vi "StatisticsFromArray.vi"(6 "Naverage":i32, 9 "input Ptot":dbl, 10 "input VAR":dbl[][](array[numeric]), 11 "Stat Vars":T1) -> (0 "STD":dbl[][](graph), 1 "MU":dbl[][](graph), 3 "VAR(n+1)":T1, 5 "std":dbl, 7 "mu":dbl)   [LabVIEW 2018, in "statistics.lvlib"]
uses:
  statistics.lvlib
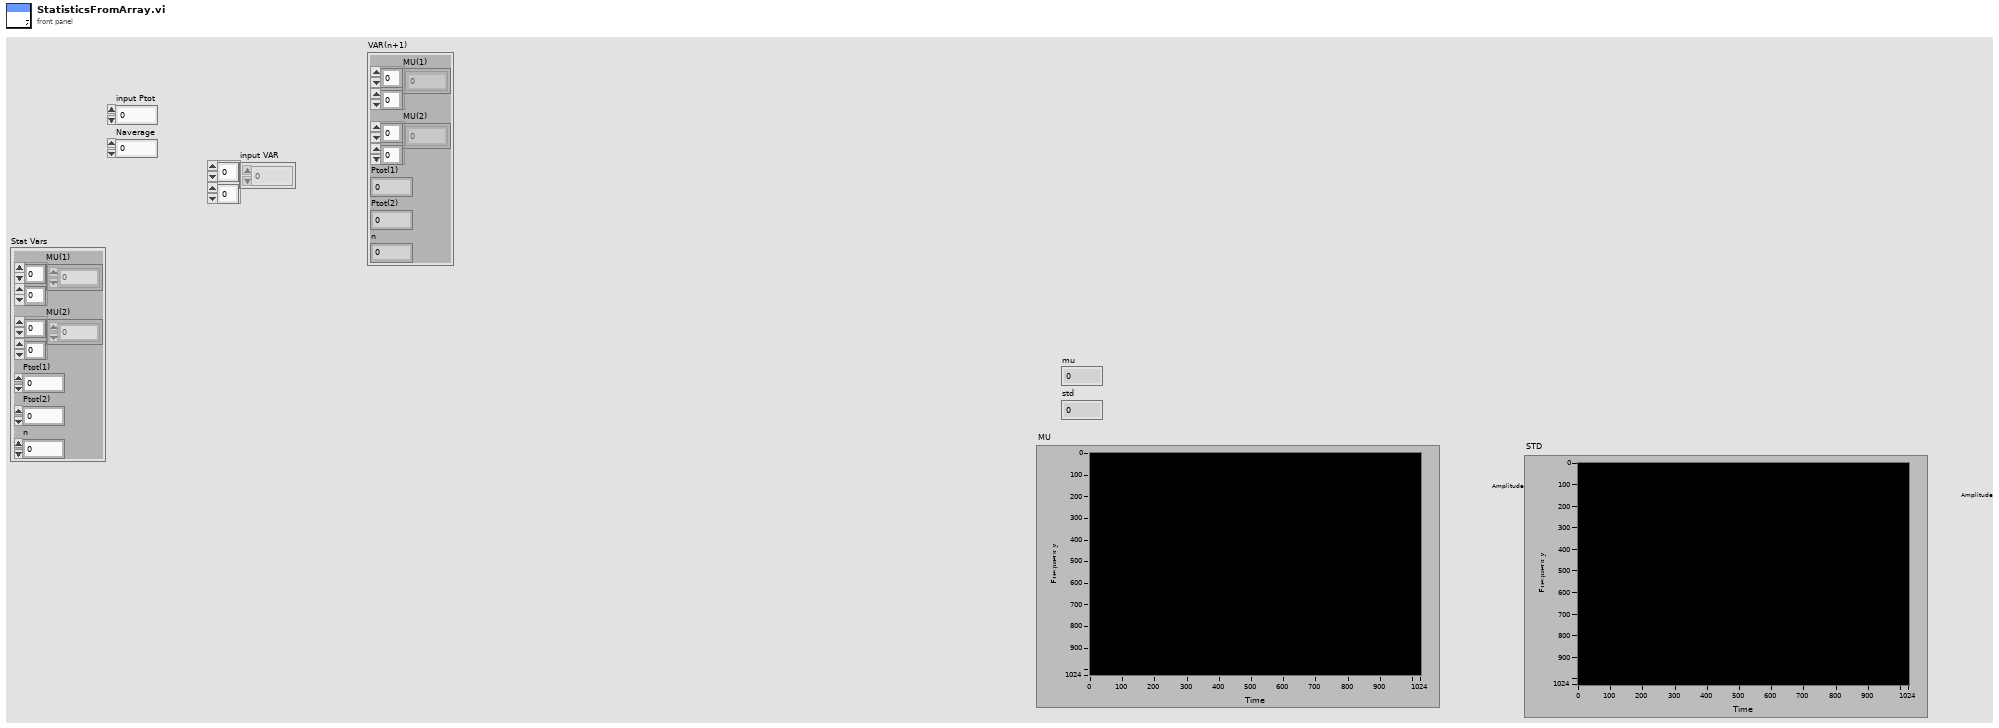
[diagram p1: front panel]
types:
  T1 = cluster{"MU(1)":dbl[][], "MU(2)":dbl[][], "Ptot(1)":dbl, "Ptot(2)":dbl, "n":i32}
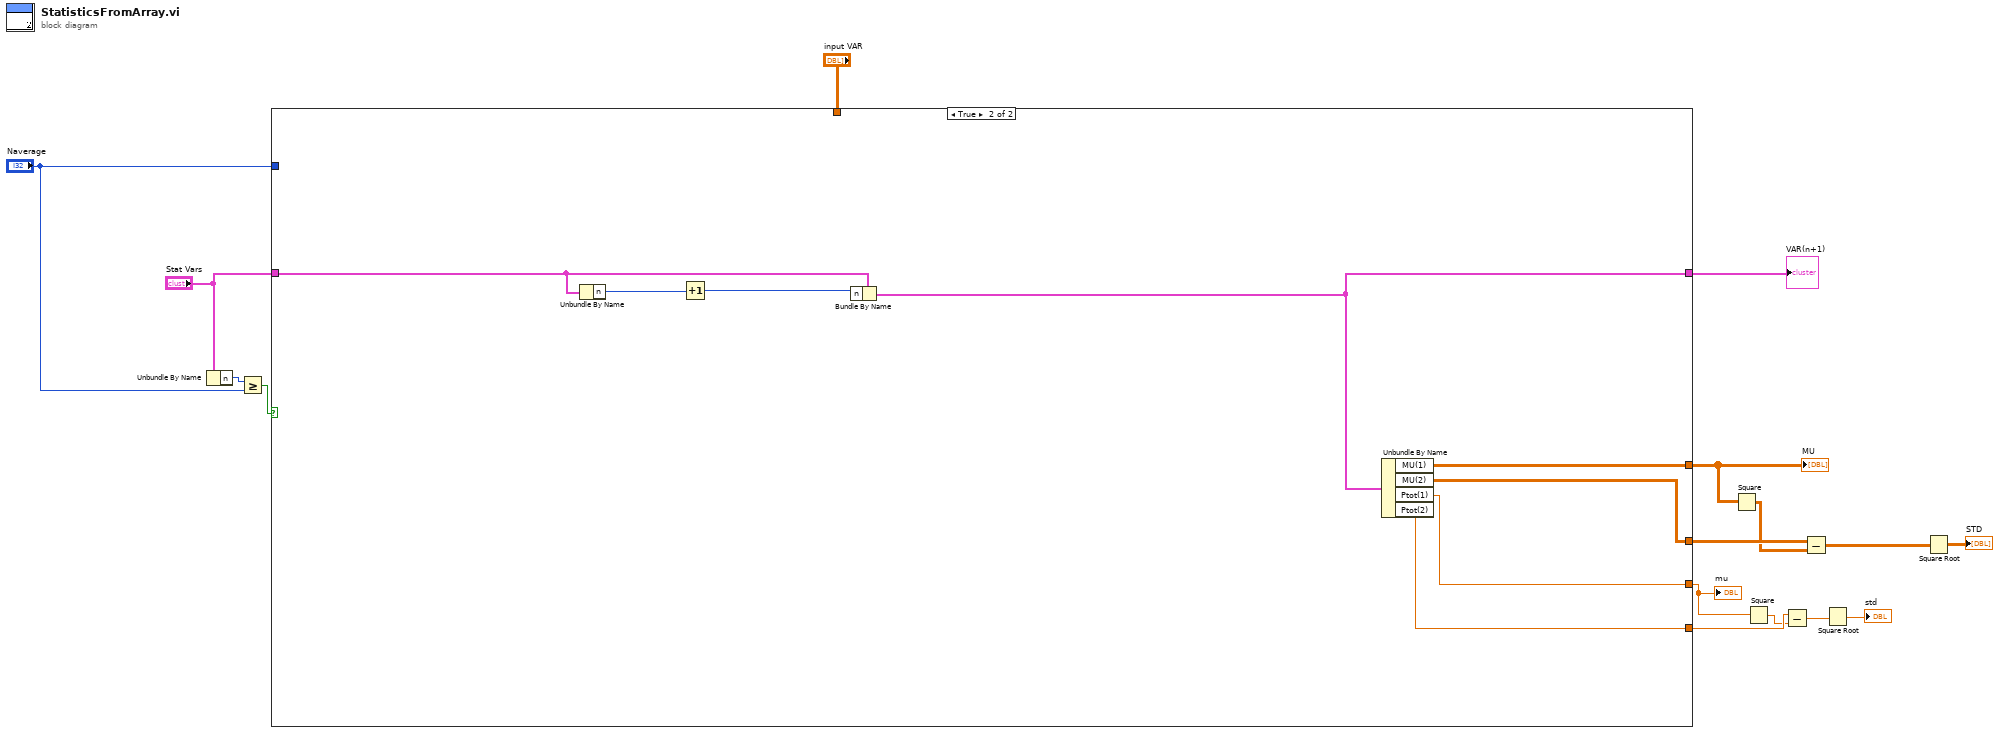
[diagram p0: block diagram]
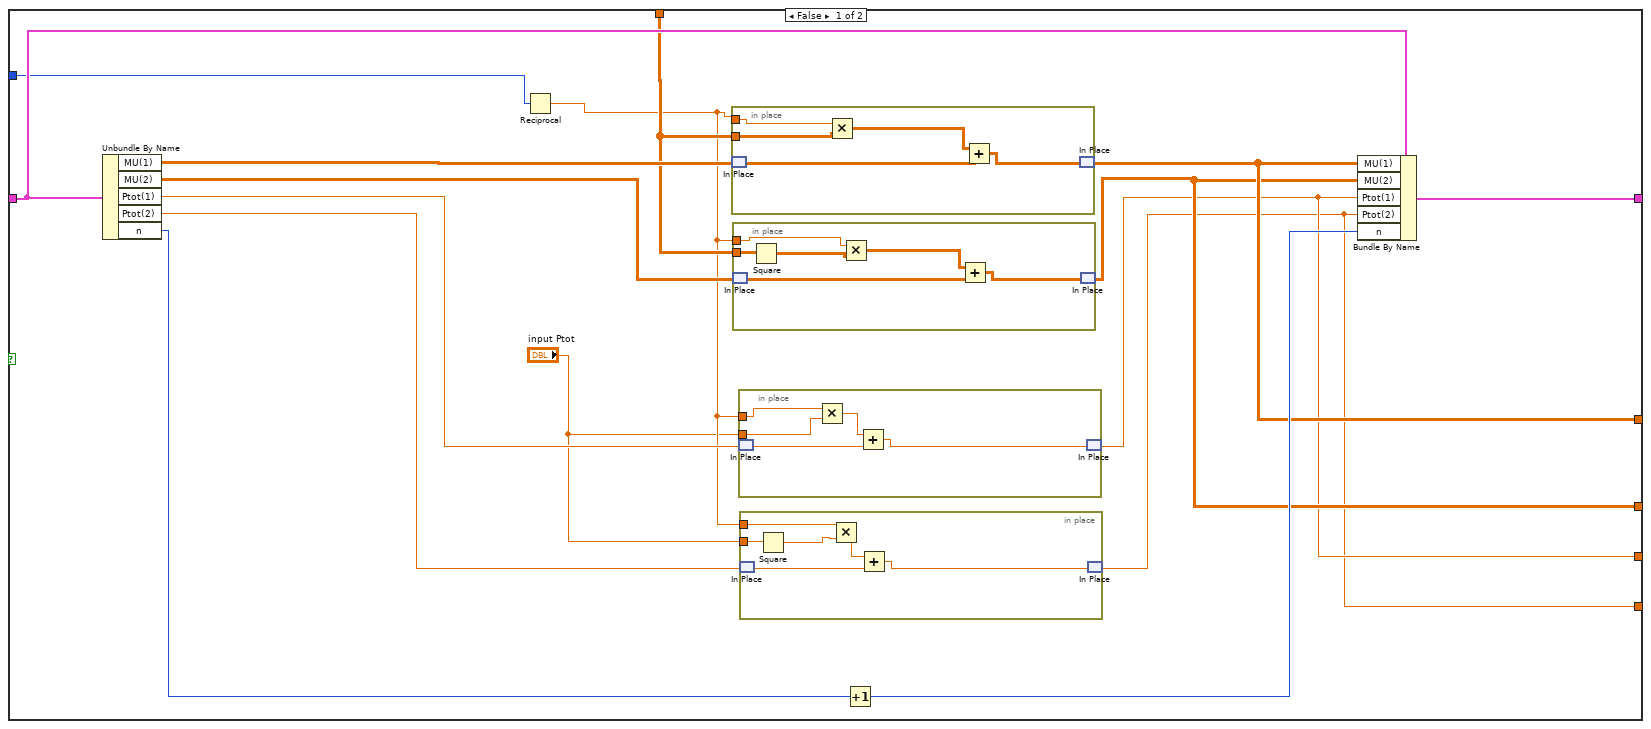
[diagram p2: hidden frame]
diagram:
  n1 = Unbundle By Name("Stat Vars") -> ("n"=w8:i32)
  n2 = Greater Or Equal?(x=w8, y="Naverage") -> (x >= y?=w6:bool)
  n3 = case shown="True" w6 {
    tunnel: "input VAR" -> [w19 _]
    tunnel: [w28 w55] -> w15
    tunnel: [w26 w62] -> w13
    tunnel: [w25 w61] -> w12
    tunnel: "Stat Vars" -> [w24 w58]
    tunnel: "Naverage" -> [w23 _]
    tunnel: [w22 w60] -> w5
    tunnel: [w21 w59] -> w2
    frame False {
      n4 = Unbundle By Name(w24) -> ("MU(1)"=w32:dbl[][], "MU(2)"=w31:dbl[][], "Ptot(1)"=w30:dbl, "Ptot(2)"=w29:dbl, "n"=w20:i32)
      n5 = Reciprocal(x=w23) -> (1/x=w18:dbl)
      n6 = in-place {
        in-place-border: w19 -> [w52]
        in-place-border: w18 -> [w51]
        n7 = in-place-match #1(w32) -> (w54:dbl[][])
        n8 = Multiply(x=w51, y=w52) -> (x*y=w50:dbl[][])
        n9 = Add(x=w50, y=w54) -> (x+y=w53:dbl[][])
        n10 = in-place-match #1(w53) -> (w26:dbl[][])
      }
      n11 = in-place {
        in-place-border: w19 -> [w47]
        in-place-border: w18 -> [w45]
        n12 = in-place-match #2(w31) -> (w49:dbl[][])
        n13 = Square(x=w47) -> (x^2=w46:dbl[][])
        n14 = Multiply(x=w45, y=w46) -> (x*y=w44:dbl[][])
        n15 = Add(x=w44, y=w49) -> (x+y=w48:dbl[][])
        n16 = in-place-match #2(w48) -> (w25:dbl[][])
      }
      n17 = in-place {
        in-place-border: "input Ptot" -> [w41]
        in-place-border: w18 -> [w40]
        n18 = in-place-match #3(w30) -> (w43:dbl)
        n19 = Multiply(x=w40, y=w41) -> (x*y=w39:dbl)
        n20 = Add(x=w39, y=w43) -> (x+y=w42:dbl)
        n21 = in-place-match #3(w42) -> (w22:dbl)
      }
      n22 = in-place {
        in-place-border: "input Ptot" -> [w36]
        in-place-border: w18 -> [w35]
        n23 = in-place-match #4(w29) -> (w38:dbl)
        n24 = Square(x=w36) -> (x^2=w34:dbl)
        n25 = Multiply(x=w35, y=w34) -> (x*y=w33:dbl)
        n26 = Add(x=w33, y=w38) -> (x+y=w37:dbl)
        n27 = in-place-match #4(w37) -> (w21:dbl)
      }
      n28 = Increment(x=w20) -> (x+1=w27:i32)
      n29 = Bundle By Name(cluster=w24, "MU(1)"=w26, "MU(2)"=w25, "Ptot(1)"=w22, "Ptot(2)"=w21, "n"=w27) -> (w28:T1)
    }
    frame True {
      n30 = Unbundle By Name(w58) -> ("n"=w57:i32)
      n31 = Increment(x=w57) -> (x+1=w56:i32)
      n32 = Bundle By Name(cluster=w58, "n"=w56) -> (w55:T1)
      n33 = Unbundle By Name(w55) -> ("MU(1)"=w62:dbl[][], "MU(2)"=w61:dbl[][], "Ptot(1)"=w60:dbl, "Ptot(2)"=w59:dbl)
    }
  }
  "VAR(n+1)" <- w15
  "MU" <- w13
  "mu" <- w5
  n34 = Square(x=w13) -> (x^2=w11:dbl[][])
  n35 = Square(x=w5) -> (x^2=w1:dbl)
  n36 = Subtract(x=w2, y=w1) -> (x-y=w4:dbl)
  n37 = Subtract(x=w12, y=w11) -> (x-y=w10:dbl[][])
  n38 = Square Root(x=w4) -> (sqrt(x)=→"std":dbl)
  n39 = Square Root(x=w10) -> (sqrt(x)=→"STD":dbl[][])
